vi "Initialize Chromosome.vi"(7 "# of Genes":u32, 8 "error in":errorcluster, 11 "Gene Type In":refnum<class "IGene.lvclass">) -> (0 "error out":errorcluster, 3 "Chromosome out":refnum<class "IChromosome.lvclass">)   [LabVIEW 2016, in "IChromosome.lvclass"]
uses:
  IChromosome.lvclass
  IGene/IGene.lvclass
  IChromosome.lvclass/IChromosome.ctl
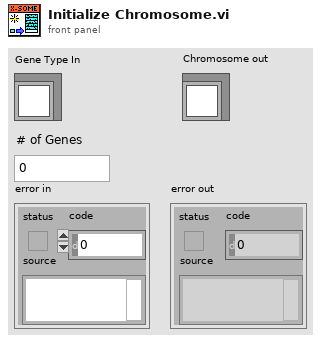
[diagram p1: front panel]
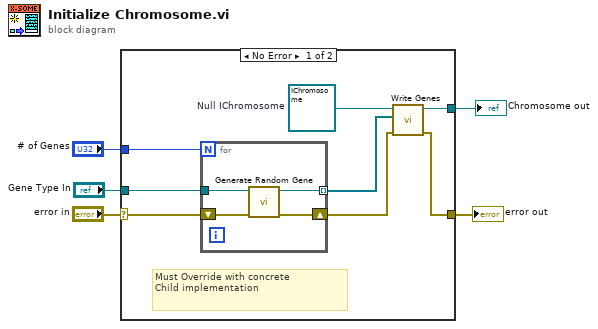
[diagram p0: block diagram]
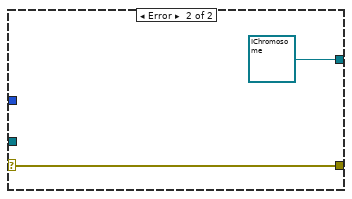
[diagram p2: hidden frame]
diagram:
  n1 = case shown="No Error" "error in" {
    selector: "error in" -> [w9 w19]
    tunnel: [w7 w19] -> w4
    tunnel: [w13 refnum<class "IChromosome.lvclass"> refnum ("IChromosome out")] -> w3
    tunnel: "# of Genes" -> [w12 _]
    tunnel: "Gene Type In" -> [w10 _]
    frame No Error {
      w6 = refnum<class "IChromosome.lvclass"> refnum  # Null IChromosome
      # "Must Override with concrete\nChild implementation"
      n2 = for {
        N: w12 -> [_]
        tunnel: [w17] -> w11 mode=indexing
        tunnel: w10 -> [w16]
        shift-right: [w14] -> w8
        shift-left: w9 -> [w15]
        n3 = call-dynamic "Generate Random Gene.vi"("error in"=w15, "IGene in"=w16) -> ("error out"=w14:errorcluster, "IGene out"=w17:refnum<class "IGene.lvclass">)  [unwired: 8 in]
      }
      n4 = call "Write Genes.vi"("error in"=w8, "Genes"=w11, "IChromosome in"=w6) -> ("error out"=w7:errorcluster, "IChromosome out"=w13:refnum<class "IChromosome.lvclass">)  [unwired: 7 in]
    }
    frame Error {
    }
  }
  "error out" <- w4
  "Chromosome out" <- w3
